vi "Intake.vi"(10 "Intake State":enum16{"neutral", "rotate", "intake", "eject"}(ring), 11 "Intake":bool) -> ()   [LabVIEW 2014]
uses:
  <vilib>/Rock Robotics/WPI/Solenoid/WPI_SolenoidValue.ctl
  <vilib>/Rock Robotics/WPI/Solenoid/WPI_SolenoidGetEnum.vi
  <vilib>/Rock Robotics/WPI/Solenoid/WPI_SolenoidSetEnum.vi
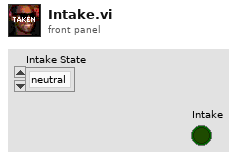
[diagram p1: front panel]
types:
  T1 = typedef "WPI_SolenoidValue.ctl" = enum16{"Off", "On", "Forward", "Reverse"}
  T2 = typedef "WPI_SolenoidDevRef.ctl" = cluster{"DevStatus":errorcluster, "Pneumatics Control Module":u8, "Forward Solenoid Channel":T3, "Reverse Solenoid Channel":T3}
  T3 = typedef "WPI_SolenoidChannel.ctl" = enum8{"Solenoid 0", "Solenoid 1", "Solenoid 2", "Solenoid 3", "Solenoid 4", "Solenoid 5", "Solenoid 6", "Solenoid 7", "Invalid"}
  T4 = typedef "WPI_MotorControlDeviceRef.ctl" = cluster{"DeviceStatus":errorcluster, "Type":T5, "PWM":cluster{"Controller":T6, "PWM Channel":T7, "DeadBand":T8}, "CAN":cluster{"Device Number":u8, "Control Mode":T9, "Semaphore":T10, "Max Vout":dbl, "TalonSRX Control Mode":T11}, "Invert":bool, "TransformRef":T12, "InvTransformRef":T12}
  T5 = typedef "WPI_MotorControlType.ctl" = enum16{"PWM", "CAN", "CANTalonSRX"}
  T6 = typedef "FPGA_TypedefDigitalModule.ctl" = enum16{"Controller 1"}
  T7 = typedef "FPGA_DIOPWMChannel.ctl" = enum8{"PWM 0", "PWM 1", "PWM 2", "PWM 3", "PWM 4", "PWM 5", "PWM 6", "PWM 7", "PWM 8", "PWM 9", "PWM MXP 0", "PWM MXP 1", "PWM MXP 2", "PWM MXP 3", "PWM MXP 4", "PWM MXP 5", "PWM MXP 6", "PWM MXP 7", "PWM MXP 8", "PWM MXP 9", "Invalid"}
  T8 = typedef "WPI_PWMDeadband.ctl" = cluster{"Name":string, "maxPositivePwm":i32, "minPositivePwm":i32, "centerPwm":i32, "maxNegativePwm":i32, "minNegativePwm":i32, "angularRange":u16}
  T9 = typedef "WPI_CANJaguar_ControlMode.ctl" = enum8{"Percent VBus", "Current", "Speed", "Position", "Voltage"}
  T10 = typedef "Semaphore RefNum" = refnum<k1>
  T11 = typedef "WPI_CANTalonSRX_APIControlMode.ctl" = enum8{"Percent VBus", "Speed", "Position", "Slave", "Unchanged / Invalid"}
  T12 = typedef "WPI_PWMTransform_ConPane.ctl" = refnum<vi>
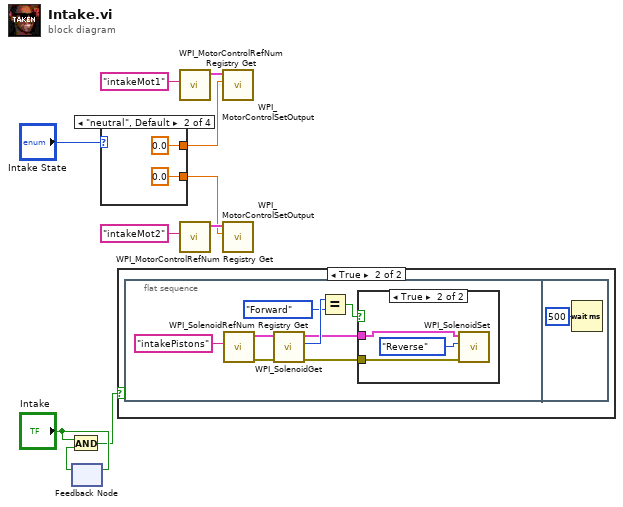
[diagram p0: block diagram]
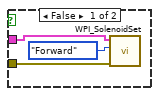
[diagram p3: hidden frame]
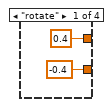
[diagram p4: hidden frame]
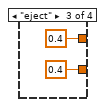
[diagram p5: hidden frame]
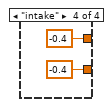
[diagram p6: hidden frame]
diagram:
  n1 = feedback-in #1("Intake") -> ()
  n2 = feedback #1() -> (w2:bool)  [unwired: 1 in]
  n3 = And(x="Intake", y=w2) -> (x .and. y?=w1:bool)
  n4 = case shown="\"neutral\", Default" "Intake State" {
    tunnel: [0.4 ("Output") 0.0 ("Output") 0.4 ("Output") -0.4 ("Output")] -> w6
    tunnel: [-0.4 ("Output") 0.0 ("Output") 0.4 ("Output") -0.4 ("Output")] -> w5
    frame "rotate" {
    }
    frame "neutral", Default {
    }
    frame "eject" {
    }
    frame "intake" {
    }
  }
  n5 = case shown="True" w1 {
    frame False {
    }
    frame True {
      n6 = flat-sequence {
        frame #0 {
          n7 = call <vilib>:"WPI_SolenoidRefNum Registry Get.vi"("refnum name"="intakePistons") -> ("error out"=w24:errorcluster, "SolenoidDevRef"=w25:T2)  [unwired: 9 in]
          n8 = call-poly <vilib>:"WPI_SolenoidGet.vi"("error in (no error)"=w24, "SolenoidDevRef"=w25) -> ("error out"=w19:errorcluster, "Value"=w23:T1, "SolenoidDevRef"=w20:T2)  [unwired: 7 in]
          n9 = Equal?(x=w23, y=WPI_SolenoidValue."Forward") -> (x = y?=w21:bool)
          n10 = case shown="True" w21 {
            tunnel: w20 -> [w28 w31]
            tunnel: w19 -> [w27 w30]
            frame False {
              n11 = call-poly <vilib>:"WPI_SolenoidSet.vi"("error in (no error)"=w27, "Value"=WPI_SolenoidValue."Forward", "SolenoidDevRef"=w28) -> ()  [unwired: 7 in, 2 out]
            }
            frame True {
              n12 = call-poly <vilib>:"WPI_SolenoidSet.vi"("error in (no error)"=w30, "Value"=WPI_SolenoidValue."Reverse", "SolenoidDevRef"=w31) -> ()  [unwired: 7 in, 2 out]
            }
          }
        }
        frame #1 {
          n13 = Wait (ms)(milliseconds to wait=u32 500) -> ()  [unwired: 1 out]
        }
      }
    }
  }
  n14 = call <vilib>:"WPI_MotorControlRefNum Registry Get.vi"("refnum name"="intakeMot1") -> ("MotorControlDevRef"=w9:T4)  [unwired: 9 in, 1 out]
  n15 = call <vilib>:"WPI_MotorControlRefNum Registry Get.vi"("refnum name"="intakeMot2") -> ("MotorControlDevRef"=w10:T4)  [unwired: 9 in, 1 out]
  n16 = call <vilib>:"WPI_MotorControlSetOutput.vi"("Output"=w6, "MotorControlDevRef"=w9) -> ()  [unwired: 7 in, 3 out]
  n17 = call <vilib>:"WPI_MotorControlSetOutput.vi"("Output"=w5, "MotorControlDevRef"=w10) -> ()  [unwired: 7 in, 3 out]
